vi "Get Anchor Coordinates ByRef.vi"(8 "error in (no error)":errorcluster, 10 "Raw Coords":cluster{"X":i32, "Y":i32}, 11 "Shape Ref":refnum<data-value>) -> (0 "error out":errorcluster, 2 "Anchor Coords":cluster{"X":i32, "Y":i32}, 3 "Shape Ref 2":refnum<data-value>)   [LabVIEW 2017, in "LV Image Editor Framework.lvlib" / "Shape.lvclass"]
uses:
  <vilib>/LIEF/Forms/Shape/Shape.lvclass
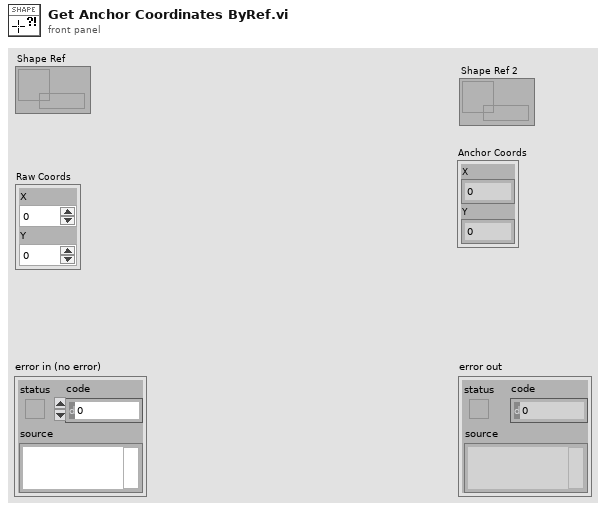
[diagram p1: front panel]
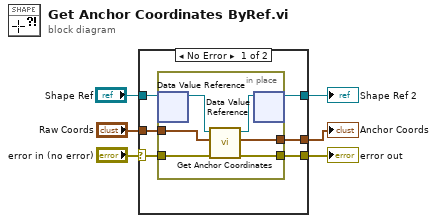
[diagram p0: block diagram]
diagram:
  n1 = case shown="No Error" "error in (no error)" {
    selector: "error in (no error)" -> [w9 w20]
    tunnel: [w8 w20] -> w5
    tunnel: [w10 w19] -> w2
    tunnel: "Shape Ref" -> [w11 w19]
    tunnel: [w12 _] -> w3
    tunnel: "Raw Coords" -> [w7 _]
    frame No Error {
      n2 = in-place {
        in-place-border: [w16] -> w12
        in-place-border: w9 -> [w15]
        in-place-border: [w14] -> w8
        in-place-border: w7 -> [w13]
        n3 = in-place-dvr #1(w11) -> (w18:refnum<class "Shape.lvclass">)  [unwired: 1 out]
        n4 = call-dynamic "Get Anchor Coordinates.vi"("error in (no error)"=w15, "Raw Coords"=w13, "Shape in"=w18) -> ("error out"=w14:errorcluster, "Anchor Coords"=w16:cluster{dbl, dbl}, "Shape out"=w17:refnum<class "Shape.lvclass">)  [unwired: 6 in]
        n5 = in-place-dvr #1(w17) -> (w10:refnum<data-value>)  [unwired: 1 out]
      }
    }
    frame Error {
    }
  }
  "error out" <- w5
  "Anchor Coords" <- w3
  "Shape Ref 2" <- w2
